vi "Get Variable.vi"(8 "error in (no error)":errorcluster, 10 "Name":string, 11 "Execution in":refnum<data-value>) -> (0 "error out":errorcluster, 2 "Value":variant, 3 "Execution out":refnum<data-value>)   [LabVIEW 2015, in "Execution.lvclass"]
uses:
  Execution.lvclass
  Project.lvclass
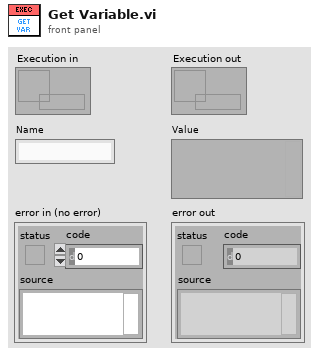
[diagram p1: front panel]
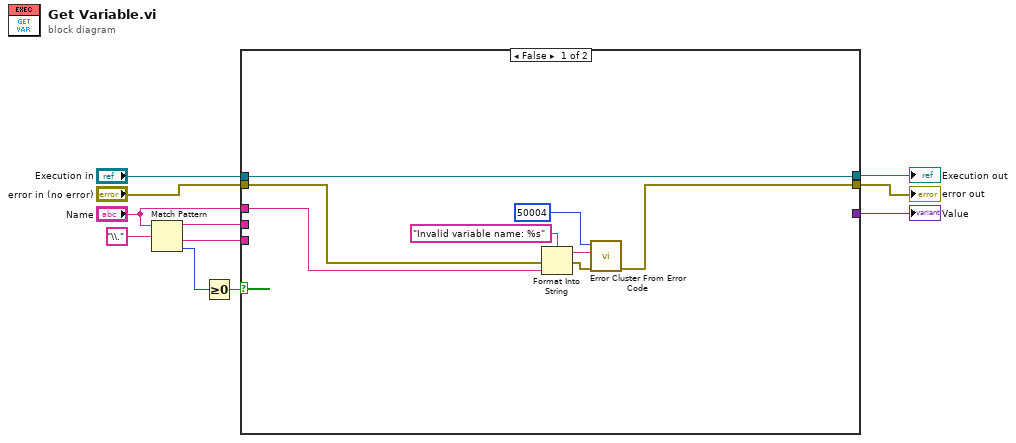
[diagram p0: block diagram]
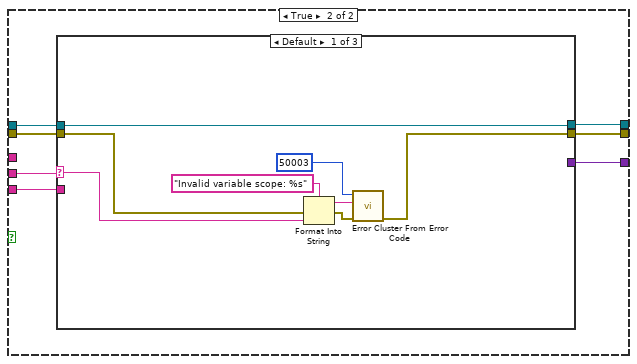
[diagram p2: hidden frame]
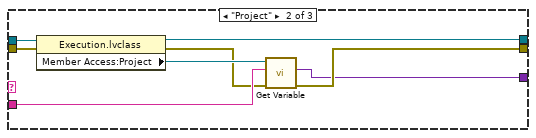
[diagram p3: hidden frame]
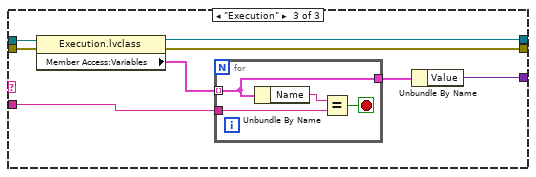
[diagram p4: hidden frame]
diagram:
  n1 = Match Pattern(string="Name", regular expression="\\.") -> (before substring=w7:string, after substring=w8:string, offset past match=w10:i32)  [unwired: 1 in, 1 out]
  n2 = Greater Or Equal To 0?(x=w10) -> (x >= 0?=w9:bool)
  n3 = case shown="False" w9 {
    tunnel: w8 -> [_ w24]
    tunnel: w7 -> [_ w26]
    tunnel: "Execution in" -> [w15 w25]
    tunnel: "error in (no error)" -> [w14 w23]
    tunnel: [_ w22] -> w4
    tunnel: [w15 w21] -> w3
    tunnel: [w12 w20] -> w2
    tunnel: "Name" -> [w13 _]
    frame False {
      n4 = Format Into String(format string="Invalid variable name: %s" ("error message (\"\")"), error in=w14, w13) -> (resulting string=w18:string, error out=w17:errorcluster)  [unwired: 1 in]
      n5 = call <vilib>:"Error Cluster From Error Code.vi"("error in (no error)"=w17, "error message (\"\")"=w18, "error code (0)"=50004) -> ("error out"=w12:errorcluster)  [unwired: 6 in]
    }
    frame True {
      n6 = case shown="Default" w26 {
        selector: w26 -> [w28 _ _]
        tunnel: w25 -> [w34 w42 w50]
        tunnel: w24 -> [_ w40 w48]
        tunnel: w23 -> [w29 w39 w49]
        tunnel: [_ w36 w45] -> w22
        tunnel: [w34 w35 w44] -> w21
        tunnel: [w27 w37 w43] -> w20
        frame Default {
          n7 = Format Into String(format string="Invalid variable scope: %s" ("error message (\"\")"), error in=w29, w28) -> (resulting string=w32:string, error out=w31:errorcluster)  [unwired: 1 in]
          n8 = call <vilib>:"Error Cluster From Error Code.vi"("error in (no error)"=w31, "error message (\"\")"=w32, "error code (0)"=50003) -> ("error out"=w27:errorcluster)  [unwired: 6 in]
        }
        frame "Project" {
          n9 = property class="Execution.lvclass"(reference=w42, error in=w39) -> (reference out=w35:refnum<data-value>, error out=w38:errorcluster, "Member Access:Project"=w41:refnum<class "Project.lvclass">)
          n10 = call-dynamic "Get Variable.vi"("error in (no error)"=w38, "Name"=w40, "Project in"=w41) -> ("error out"=w37:errorcluster, "Value"=w36:variant)  [unwired: 6 in, 1 out]
        }
        frame "Execution" {
          n11 = property class="Execution.lvclass"(reference=w50, error in=w49) -> (reference out=w44:refnum<data-value>, error out=w43:errorcluster, "Member Access:Variables"=w47:cluster{"Name":string, "Value":variant}[])
          n12 = for {
            tunnel: w48 -> [w53]
            tunnel: w47 -> [w52] mode=indexing
            tunnel: [w52] -> w46
            stop <- w51 stop-if-true
            n13 = Unbundle By Name(w52) -> ("Name"=w54:string)
            n14 = Equal?(x=w54, y=w53) -> (x = y?=w51:bool)
          }
          n15 = Unbundle By Name(w46) -> ("Value"=w45:variant)
        }
      }
    }
  }
  "error out" <- w2
  "Value" <- w4
  "Execution out" <- w3
